vi "Periodic Tasks.vi"(8 "error in":errorcluster) -> ()   [LabVIEW 2017]
doc: "This VI runs in parallel to other robot code. It can contain as many user-defined periodic loops as you need. These can carry out PID or other sorts of timed response."
uses:
  <vilib>/Rock Robotics/WPI/Utilities/WPI_GetSetVariantRefNum.vi
  Robot Global Data.vi
panel:
  out "Angle":dbl(knob) scale=0.0..360.0
  in  "Reset Zero Position":bool
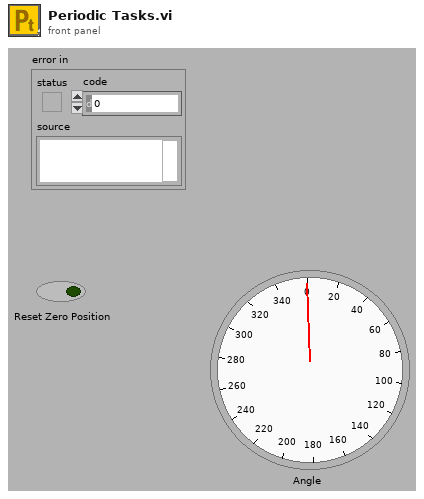
[diagram p1: front panel]
types:
  T1 = typedef "WPI_JoystickDevRef.ctl" = cluster{"Device":T2}
  T2 = typedef "WPI_JoystickDeviceEnum.ctl" = enum16{"USB 0", "USB 1", "USB 2", "USB 3", "USB 4", "USB 5"}
  T3 = typedef "WPI_GyroDevRef.ctl" = cluster{"DevStatus":errorcluster, "Analog Channel":T4, "Gain (VoltsPerDegree/Second)":dbl, "Gyro Type":enum16{"Analog", "XRS450"}, "Handle":i32, "SPI Bus":T5, "Device Found":bool, "Sample Rate":dbl, "Calibrate On Open":bool, "Offset":dbl}
  T4 = typedef "FPGA_AIChannel.ctl" = enum8{"AI 0", "AI 1", "AI 2", "AI 3", "AI MXP 0", "AI MXP 1", "AI MXP 2", "AI MXP 3", "Invalid"}
  T5 = typedef "spi_bus.ctl" = enum16{"SPI On-Board, CS0", "SPI On-Board, CS1", "SPI On-Board, CS2", "SPI On-Board, CS3", "SPI MXP", "Invalid"}
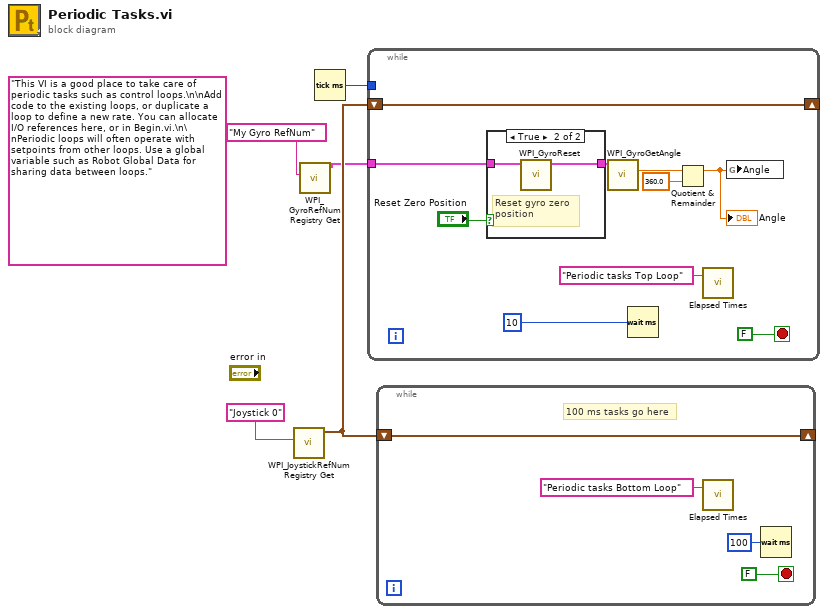
[diagram p0: block diagram]
diagram:
  (unwired) "This VI is a good place to take care of periodic tasks such as control loops.\n\nAdd code to the existing loops, or duplicate a loop to define a new rate. You can allocate I/O references here, or in Begin.vi.\n\nPeriodic loops will often operate with setpoints from other loops. Use a global variable such as Robot Global Data for sharing data between loops."
  n1 = call <vilib>:"WPI_JoystickRefNum Registry Get.vi"("refnum name"="Joystick 0") -> ("JoystickDevRef"=w4:T1)  [unwired: 1 in, 9 out]
  n2 = call <vilib>:"WPI_GyroRefNum Registry Get.vi"("refnum name"="My Gyro RefNum") -> ("GyroDevRef"=w2:T3)  [unwired: 9 in, 1 out]
  n3 = Tick Count (ms)() -> (millisecond timer value=w3:u32)
  n4 = while {
    shift-right: [w14] -> _
    shift-left: w4 -> [w14]
    tunnel: w3 -> [_]
    tunnel: w2 -> [w10]
    stop <- FALSE stop-if-true
    n5 = case shown="True" "Reset Zero Position" {
      tunnel: w10 -> [w16 w18]
      tunnel: [w16 w17] -> w12
      frame False {
      }
      frame True {
        # "Reset gyro zero \nposition"
        n6 = call <vilib>:"WPI_GyroReset.vi"("GyroDevRef"=w18) -> ("GyroDevRef"=w17:T3)  [unwired: 10 out]
      }
    }
    n7 = call <vilib>:"WPI_GyroGetAngle.vi"("GyroDevRef"=w12) -> ("Angle"=w8:dbl)  [unwired: 1 in, 9 out]
    n8 = Wait (ms)(milliseconds to wait=u32 10) -> ()  [unwired: 1 out]
    n9 = Quotient & Remainder(x=w8, y=360.0) -> (x-y*floor(x/y)=w7:dbl)  [unwired: 1 out]
    "Angle" <- w7
    n10 = call "Elapsed Times.vi"("Call Name"="Periodic tasks Top Loop") -> ()  [unwired: 2 in, 1 out]
    n11 = global write "Robot Global Data.vi" "Angle"(w7) -> ()
  }
  n12 = while {
    shift-right: [w20] -> _
    shift-left: w4 -> [w20]
    stop <- FALSE stop-if-true
    # "100 ms tasks go here"
    n13 = call "Elapsed Times.vi"("Call Name"="Periodic tasks Bottom Loop") -> ()  [unwired: 2 in, 1 out]
    n14 = Wait (ms)(milliseconds to wait=u32 100) -> ()  [unwired: 1 out]
  }
